vi "AlternatingLEDs.vi"() -> ()   [LabVIEW 2014]
doc: "This VI lits up two different LED's alternatingly with a wait time of 1000ms between them. The condition used for the LED is such that if the iteration of the loop is even, A lits up and if the iterations is B then B lits up."
panel:
  in  "Stop Button":bool
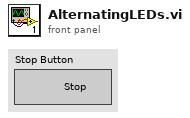
[diagram p1: front panel]
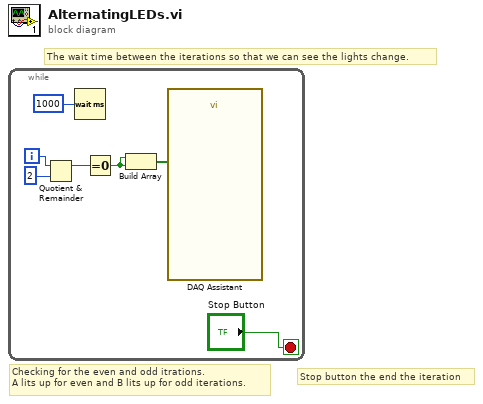
[diagram p0: block diagram]
diagram:
  # "Checking for the even and odd itrations.\nA lits up for even and B lits up for odd iterations."
  # "The wait time between the iterations so that we can see the lights change."
  # "Stop button the end the iteration"
  n1 = while {
    i -> [w6]
    stop <- "Stop Button" stop-if-true
    n2 = Quotient & Remainder(x=w6, y=2) -> (x-y*floor(x/y)=w4:i32)  [unwired: 1 out]
    n3 = Wait (ms)(milliseconds to wait=1000) -> ()  [unwired: 1 out]
    n4 = Equal To 0?(x=w4) -> (x = 0?=w1:bool)
    n5 = Build Array(w1, w1) -> (w7:bool[])
    n6 = call "DAQ Assistant"("data"=w7) -> ()  [unwired: 17 in, 2 out]
  }
